vi "Init.vi"(8 "error in (no error)":errorcluster, 10 "index":i32, 11 "BC_Evolut_1D_Numeric":refnum<class "NI_BC_Evolut_1D_Numeric.lvclass">) -> (0 "error out":errorcluster, 3 "initialized BC_Evolut_1D_Numeric":refnum<class "NI_BC_Evolut_1D_Numeric.lvclass">)   [LabVIEW 2017, in "NI_PDE.lvlib" / "NI_BC_Evolut_1D_Numeric.lvclass"]
uses:
  <vilib>/gmath/pde.llb/BCClass/BC_Evolut_1D_Numeric/NI_BC_Evolut_1D_Numeric.lvclass
  <vilib>/gmath/pde.llb/BCClass/Class Type.ctl
  <vilib>/gmath/pde.llb/Common/PDE_BC Type.ctl
  <vilib>/gmath/pde.llb/BCClass/BC_Evolut_1D_Numeric/NI_BC_Evolut_1D_Numeric.lvclass/NI_BC_Evolut_1D_Numeric.ctl
  <vilib>/gmath/pde.llb/BCClass/NI_BC.lvclass
  <vilib>/gmath/NI_PDE.lvlib
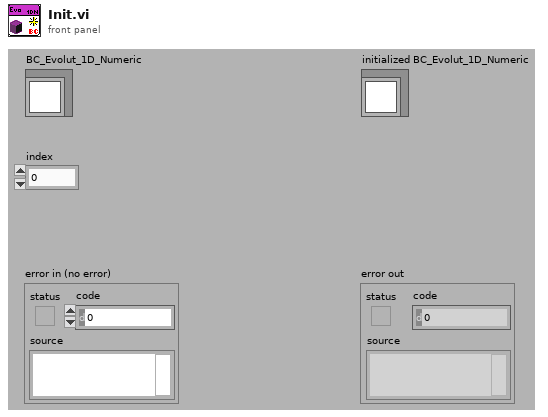
[diagram p1: front panel]
types:
  T1 = typedef "NI_PDE.lvlib/PDE_BC Type.ctl" = i32
  T2 = typedef "NI_PDE.lvlib/NI_BC.lvclass/Class Type.ctl" = i32
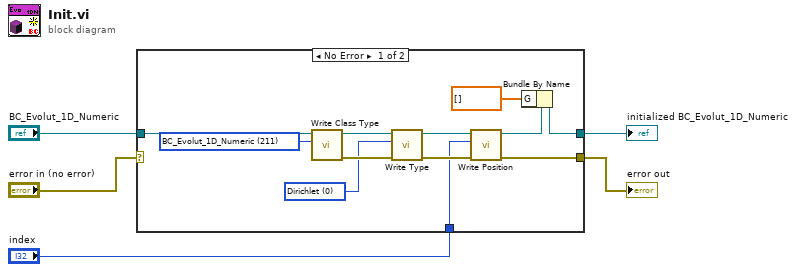
[diagram p0: block diagram]
diagram:
  n1 = case shown="No Error" "error in (no error)" {
    selector: "error in (no error)" -> [_ w18]
    tunnel: [w8 w19] -> w5
    tunnel: [w10 w18] -> w4
    tunnel: "BC_Evolut_1D_Numeric" -> [w11 w19]
    tunnel: "index" -> [w6 _]
    frame No Error {
      w12 = T1 0 items=["Dirichlet", "Neumann"] ("BC type")
      w13 = T2 211 items=["BC"=0, "BC_Steady"=100, "BC_Steady_2D"=120, "BC_Steady_2D_Numeric"=121, "BC_Steady_2D_VIRef"=122, "BC_Evolut"=200, "BC_Evolut_1D"=210, "BC_Evolut_1D_Numeric"=211, "BC_Evolut_1D_VIRef"=212, "BC_Evolut_2D"=220, "BC_Evolut_2D_Numeric"=221, "BC_Evolut_2D_VIRef"=222] ("BC class type")
      n2 = call-dynamic "Write Class Type.vi"("BC class type"=w13, "BC.lvclass in"=w11) -> ("error out"=w14:errorcluster, "BC.lvclass out"=w17:refnum<class "NI_BC_Evolut_1D_Numeric.lvclass">)  [unwired: 1 in, 7 out]
      n3 = call-dynamic "Write Type.vi"("error in (no error)"=w14, "BC type"=w12, "BC.lvclass in"=w17) -> ("error out"=w15:errorcluster, "BC.lvclass out"=w16:refnum<class "NI_BC_Evolut_1D_Numeric.lvclass">)  [unwired: 7 out]
      n4 = call-dynamic "Write Position.vi"("error in (no error)"=w15, "BC position 1D"=w6, "BC_Evolut_1D.lvclass in"=w16) -> ("error out"=w10:errorcluster, "BC_Evolut_1D.lvclass out"=w9:refnum<class "NI_BC_Evolut_1D_Numeric.lvclass">)  [unwired: 7 out]
      n5 = Bundle By Name(cluster=w9, "G"=dbl[] []) -> (w8:refnum<class "NI_BC_Evolut_1D_Numeric.lvclass">)
    }
    frame Error {
    }
  }
  "initialized BC_Evolut_1D_Numeric" <- w5
  "error out" <- w4
